vi "Mouseover.vi"(8 "error in (no error)":errorcluster, 10 "Byte Offset from Point":i32, 11 "QControlWizard in":refnum<class "QControl Creation Wizard.lvclass">) -> (0 "error out":errorcluster, 3 "QControlWizard out":refnum<class "QControl Creation Wizard.lvclass">)   [LabVIEW 2015, in "QControl Creation Wizard.lvclass"]
uses:
  QControl Creation Wizard.lvclass
  QControl Creation Wizard.lvclass/QControl Creation Wizard.ctl
  <vilib>/Utility/miscctls.llb/LVSelectionTypeDef.ctl
  <vilib>/Utility/cursorutil.llb/Set Cursor (Icon Pict).vi
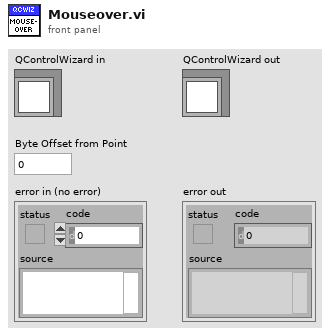
[diagram p1: front panel]
types:
  T1 = typedef "LVSelectionTypeDef.ctl" = cluster{"Selection Start":u32, "Selection End":u32}
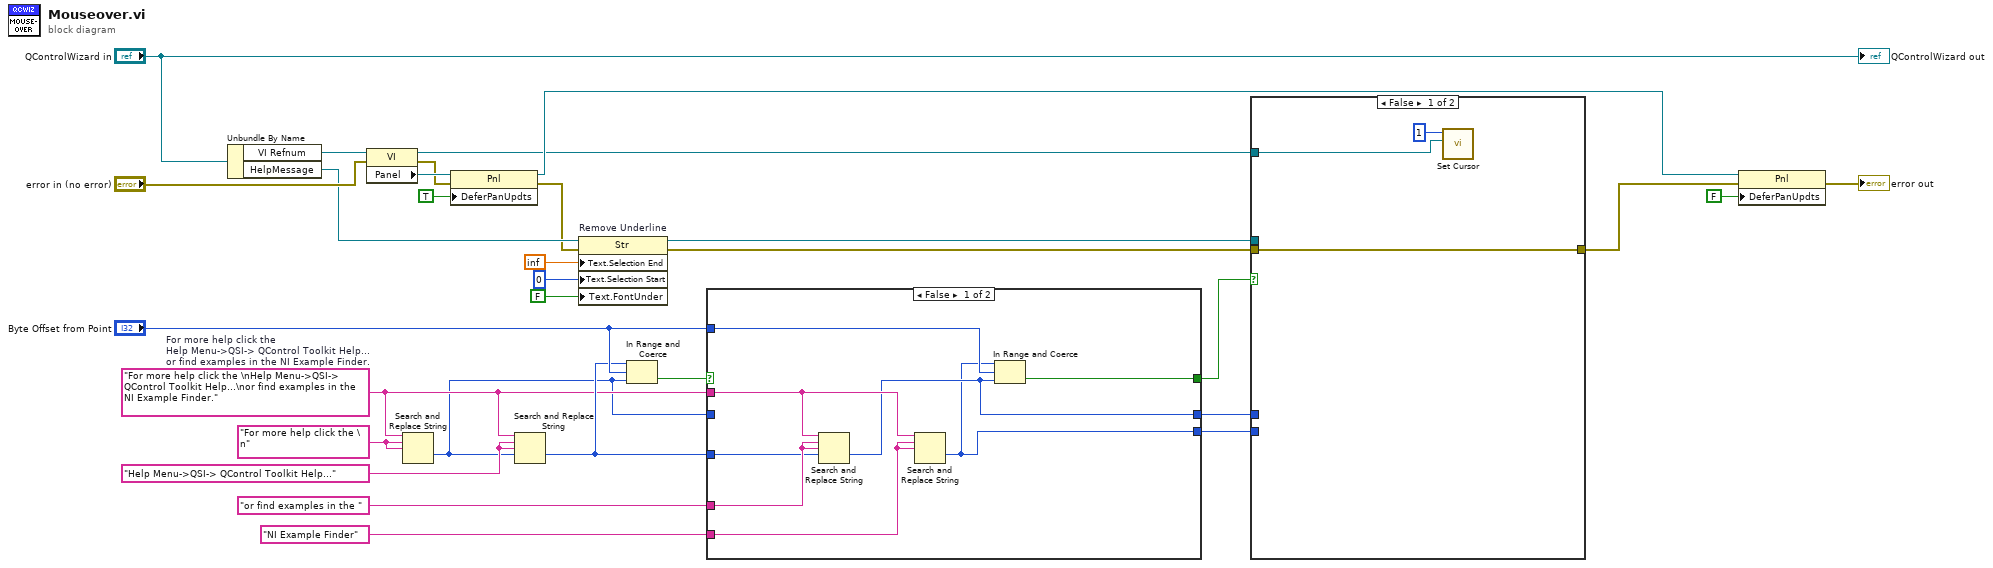
[diagram p0: block diagram]
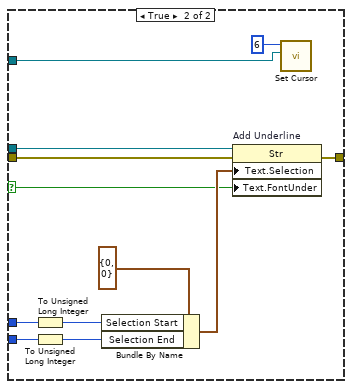
[diagram p2: hidden frame]
diagram:
  w20 = "Help Menu->QSI-> QControl Toolkit Help..."
  w24 = "For more help click the \n"
  w11 = "For more help click the \nHelp Menu->QSI-> QControl Toolkit Help...\nor find examples in the NI Example Finder."  # For more help click the  Help Menu->QSI-> QControl Toolkit Help... or find examples in the NI Example Finder.
  n1 = Unbundle By Name("QControlWizard in") -> ("VI Refnum"=w30:refnum<vi>, "HelpMessage"=w19:refnum<vi>)
  n2 = property class="VI"(reference=w30, error in="error in (no error)") -> (reference out=w2:refnum<vi>, error out=w26:errorcluster, "Panel"=w27:refnum<vi>)
  n3 = Search and Replace String(input string=w11, search string=w24, replace string=w24) -> (offset past replacement=w8:i32)  [unwired: 5 in, 3 out]
  n4 = property class="Pnl"(reference=w27, error in=w26, "DeferPanUpdts"=TRUE ("Defer Panel Updates")) -> (reference out=w22:refnum<vi>, error out=w4:errorcluster)
  n5 = Search and Replace String(input string=w11, search string=w20, replace string=w20, offset=w8) -> (offset past replacement=w12:i32)  [unwired: 4 in, 3 out]
  n6 = property on="Remove Underline" class="Str"(reference=w19, error in=w4, "Text.Selection End"=inf, "Text.Selection Start"=u32 0 ("Text.Selection:Start"), "Text.FontUnder"=FALSE ("Text.Font:Underline")) -> (reference out=w15:refnum<vi>, error out=w5:errorcluster)
  n7 = In Range and Coerce(upper limit=w12, x="Byte Offset from Point", lower limit=w8) -> (In Range?=w9:bool)  [unwired: 1 out]
  n8 = case shown="False" w9 {
    selector: w9 -> [_ w39]
    tunnel: "Byte Offset from Point" -> [w38 _]
    tunnel: "or find examples in the " -> [w37 _]
    tunnel: w12 -> [w36 w40]
    tunnel: w11 -> [w35 _]
    tunnel: "NI Example Finder" -> [w34 _]
    tunnel: w8 -> [_ w41]
    tunnel: [w33 w41] -> w7
    tunnel: [w32 w40] -> w6
    tunnel: [w31 w39] -> w1
    frame False {
      n9 = Search and Replace String(input string=w35, search string=w37, replace string=w37, offset=w36) -> (offset past replacement=w33:i32)  [unwired: 4 in, 3 out]
      n10 = Search and Replace String(input string=w35, search string=w34, replace string=w34) -> (offset past replacement=w32:i32)  [unwired: 5 in, 3 out]
      n11 = In Range and Coerce(upper limit=w32, x=w38, lower limit=w33) -> (In Range?=w31:bool)  [unwired: 1 out]
    }
    frame True {
    }
  }
  n12 = case shown="False" w1 {
    selector: w1 -> [_ w46]
    tunnel: w15 -> [_ w56]
    tunnel: w7 -> [_ w55]
    tunnel: w6 -> [_ w53]
    tunnel: w5 -> [w44 w49]
    tunnel: [w44 w48] -> w3
    tunnel: w2 -> [w42 w47]
    frame False {
      n13 = call-poly <vilib>:"Set Cursor.vi"("VI reference (current VI)"=w42, "icon"=u16 1) -> ()  [unwired: 8 in, 2 out]
    }
    frame True {
      n14 = To Unsigned Long Integer(number=w55) -> (unsigned 32bit integer=w52:u32)
      n15 = To Unsigned Long Integer(number=w53) -> (unsigned 32bit integer=w51:u32)
      n16 = Bundle By Name(cluster=T1 {"Selection Start"=0, "Selection End"=0} ("Text.Selection"), "Selection Start"=w52, "Selection End"=w51) -> (w50:T1)
      n17 = property on="Add Underline" class="Str"(reference=w56, error in=w49, "Text.Selection"=w50, "Text.FontUnder"=w46) -> (error out=w48:errorcluster)  [unwired: 1 out]
      n18 = call-poly <vilib>:"Set Cursor.vi"("VI reference (current VI)"=w47, "icon"=u16 6) -> ()  [unwired: 8 in, 2 out]
    }
  }
  n19 = property class="Pnl"(reference=w22, error in=w3, "DeferPanUpdts"=FALSE ("Defer Panel Updates")) -> (error out=→"error out":errorcluster)  [unwired: 1 out]
  "QControlWizard out" <- "QControlWizard in"
